vi "top_read_input.vi"(8 "error in (no error)":errorcluster, 10 "Dynamic data":T1, 11 "Input parameters":T2={"Measurement type"=enum."Debug", "Sensor type"=enum."HPK_8in_256", "Identifier"="test.txt", "Open after execution?"=FALSE, "Plot after execution?"=FALSE, "Display channel"=0, "Voltage Delay (s)"=0.5, "Switch Delay (s)"=0.01, "VISA resource name source"="", "VISA resource name DMM"="", "VISA resource name LCR"="", "Compliance  Level (A)"=10.0, "Voltage Limit (V)"=1000.0, "Data storage location"="", "Scan voltages"="", "Use source as DMM?"=FALSE, "LCR signal frequenzy (Hz)"=10.0, "DMM device"=enum."Keithley2001", "Sampling number"=1, "Use env. sensors on"=enum."Sensirion sht1x/7x", "Switchboard Handle"=0, "Use Switchboard"=FALSE, "LCR signal voltage (V)"=10000.0, "Repeat"=1, "Scan voltages IV"="", "Scan voltages CV"="", "Hex pad numbers?"=FALSE, "Set measurement type"=enum."Debug", "Custom pad scan"="", "IV voltage Delay (s)"=0.5, "CV voltage Delay (s)"=0.5, "Needle measurement?"=FALSE, "Comments"="test.txt", "LCR signal frequenzy (kHz)"=10.0, "Compliance  Level (uA)"=10.0, "Open Correction Array"=array2304x3[6912 elements], "Current set voltage"=0.0, "Last set voltage"=0.0, "Current channel"=0, "Last OpenCorrection index"=-1, "Total curr/vltg every x steps"=10, "Current channel iteration"=0, "No CV corrections"=FALSE, "Mapfile"="", "Corrfile"="", "IV voltage file"=path "", "CV voltage file"=path "", "IV Switch Delay (s)"=0.01, "CV Switch Delay (s)"=0.01, "Invert polarity"=FALSE, "Set debug dirs"=FALSE, "Is n on p"=FALSE} {"CV Switch Delay (s)" format="%#_13g"; "IV Switch Delay (s)" format="%#_13g"; "Last set voltage" format="%#_13g"; "Current set voltage" format="%#_13g"; "CV voltage Delay (s)" format="%#_13g"; "IV voltage Delay (s)" format="%#_13g"; "Voltage Limit (V)" format="%#_13g"; "Voltage Delay (s)" format="%#_13g"; "Switch Delay (s)" format="%#_13g"}) -> (0 "error out":errorcluster, 2 "Dynamic data":T1, 3 "Input parameters":T2={"Measurement type"=enum."Debug", "Sensor type"=enum."HPK_8in_256", "Identifier"="test.txt", "Open after execution?"=FALSE, "Plot after execution?"=FALSE, "Display channel"=0, "Voltage Delay (s)"=0.5, "Switch Delay (s)"=0.01, "VISA resource name source"="", "VISA resource name DMM"="", "VISA resource name LCR"="", "Compliance  Level (A)"=10.0, "Voltage Limit (V)"=1000.0, "Data storage location"="", "Scan voltages"="", "Use source as DMM?"=FALSE, "LCR signal frequenzy (Hz)"=10.0, "DMM device"=enum."Keithley2001", "Sampling number"=1, "Use env. sensors on"=enum."Sensirion sht1x/7x", "Switchboard Handle"=0, "Use Switchboard"=FALSE, "LCR signal voltage (V)"=10000.0, "Repeat"=1, "Scan voltages IV"="", "Scan voltages CV"="", "Hex pad numbers?"=FALSE, "Set measurement type"=enum."Debug", "Custom pad scan"="", "IV voltage Delay (s)"=0.5, "CV voltage Delay (s)"=0.5, "Needle measurement?"=FALSE, "Comments"="test.txt", "LCR signal frequenzy (kHz)"=10.0, "Compliance  Level (uA)"=10.0, "Open Correction Array"=array2304x3[6912 elements], "Current set voltage"=0.0, "Last set voltage"=0.0, "Current channel"=0, "Last OpenCorrection index"=-1, "Total curr/vltg every x steps"=10, "Current channel iteration"=0, "No CV corrections"=FALSE, "Mapfile"="", "Corrfile"="", "IV voltage file"=path "", "CV voltage file"=path "", "IV Switch Delay (s)"=0.01, "CV Switch Delay (s)"=0.01, "Invert polarity"=FALSE, "Set debug dirs"=FALSE, "Is n on p"=FALSE} {"CV Switch Delay (s)" format="%#_13g"; "IV Switch Delay (s)" format="%#_13g"; "Last set voltage" format="%#_13g"; "Current set voltage" format="%#_13g"; "CV voltage Delay (s)" format="%#_13g"; "IV voltage Delay (s)" format="%#_13g"; "Voltage Limit (V)" format="%#_13g"; "Voltage Delay (s)" format="%#_13g"; "Switch Delay (s)" format="%#_13g"})   [LabVIEW 2016]
doc: "Processes the user input to generate names and constants to be used during program execution."
uses:
  input_params.ctl
  data_dynamic.ctl
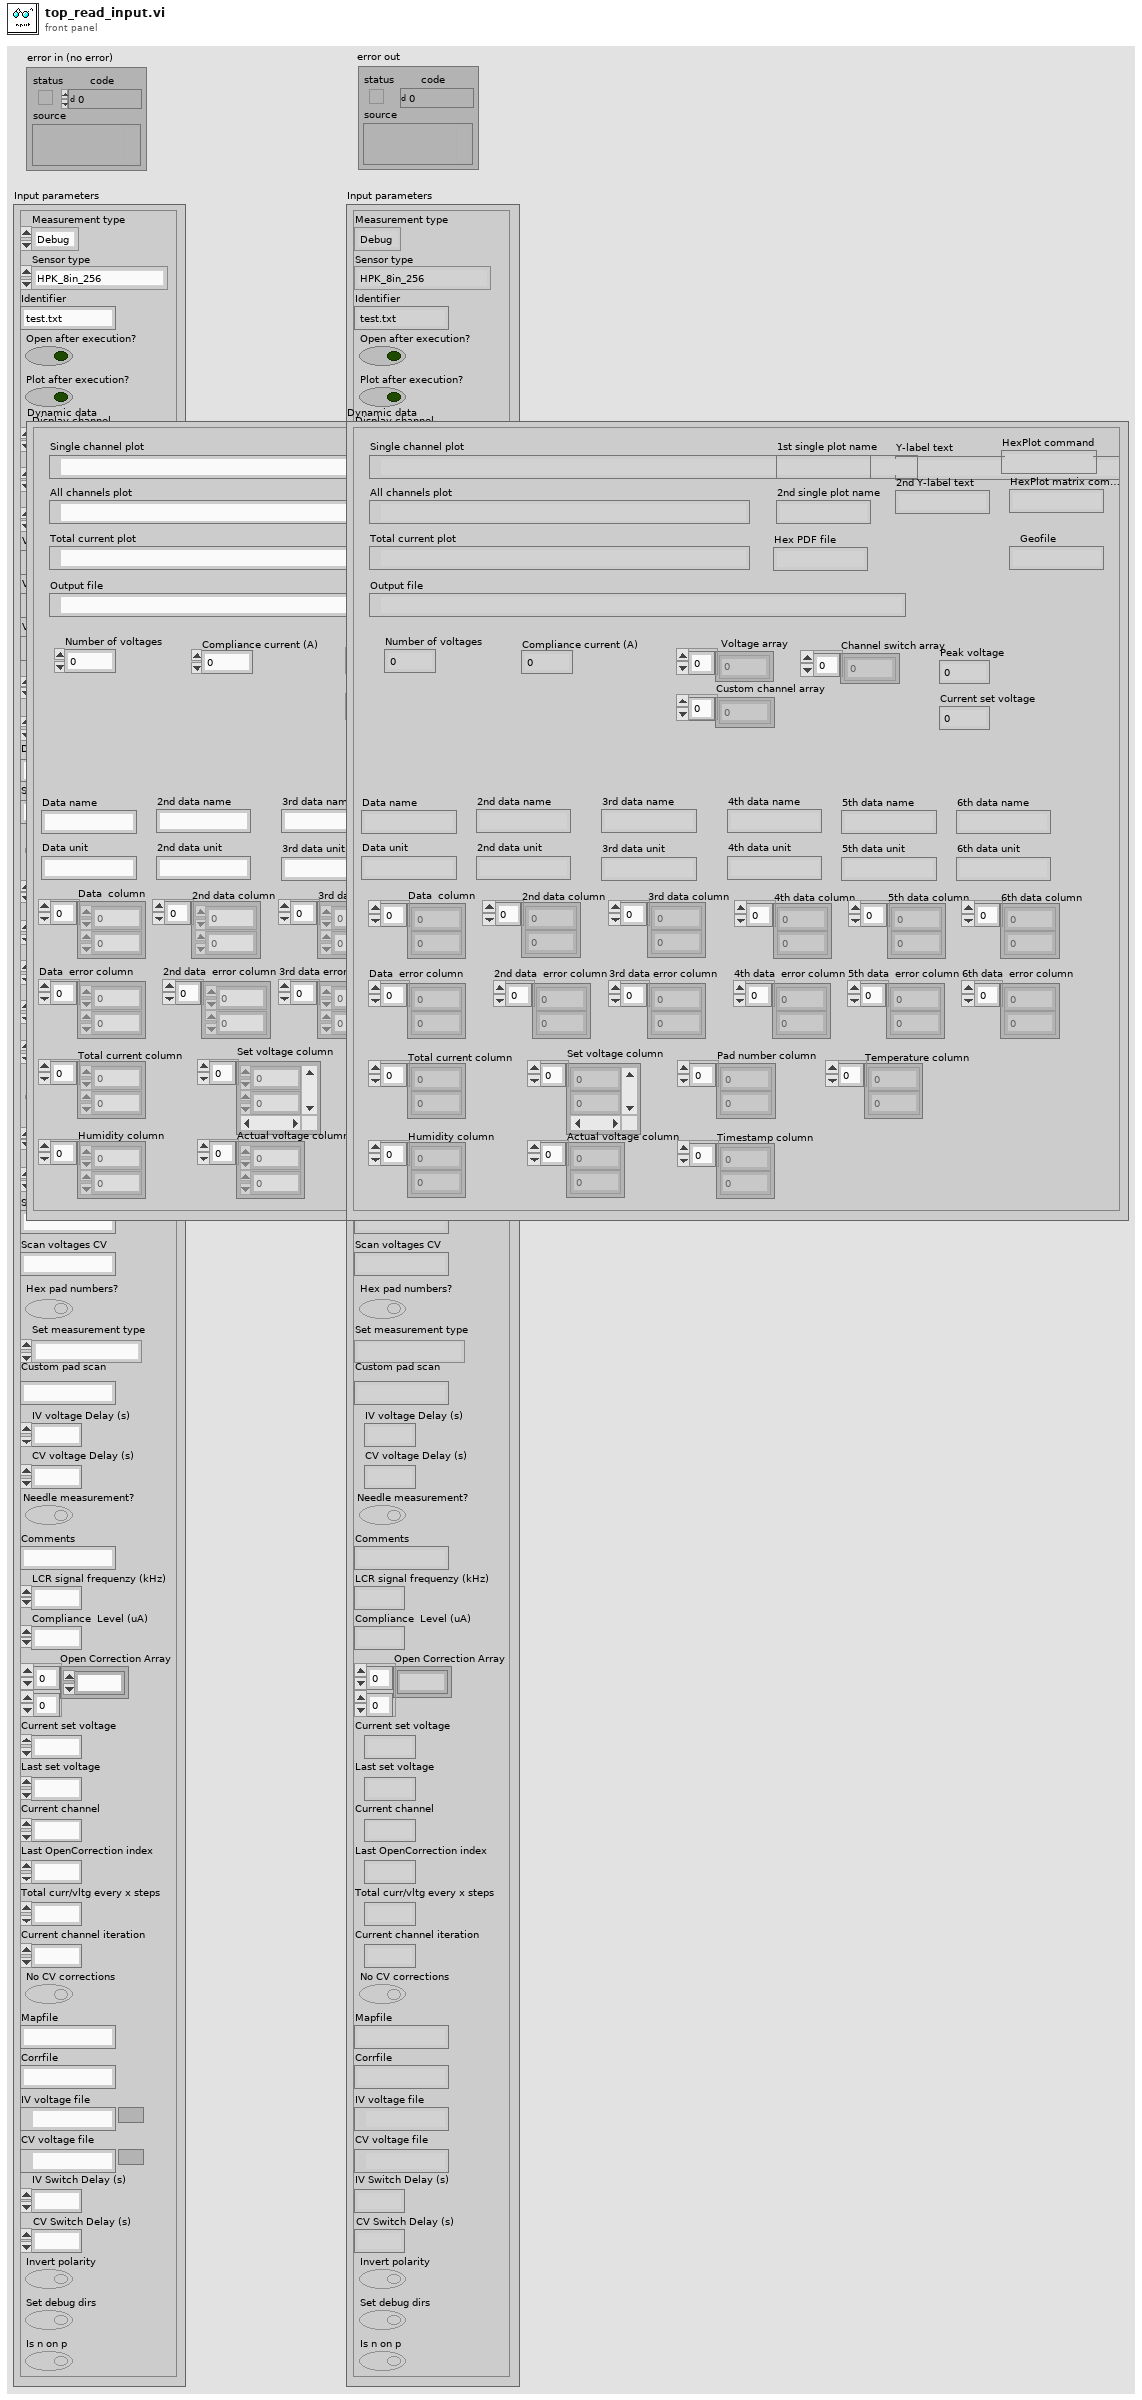
[diagram p1: front panel]
types:
  T1 = typedef "data_dynamic.ctl" = cluster{"Output file":path, "Y-label text":string, "Current set voltage":dbl, "Set voltage column":dbl[], "Pad number column":dbl[], "Data  column":dbl[], "Number of voltages":i32, "Compliance current (A)":dbl, "Geofile":string, "Peak voltage":dbl, "Hex PDF file":string, "Voltage array":dbl[], "Total current column":dbl[], "Timestamp column":dbl[], "Data name":string, "Data unit":string, "2nd data column":dbl[], "2nd data name":string, "2nd data unit":string, "3rd data column":dbl[], "4th data column":dbl[], "3rd data name":string, "3rd data unit":string, "4th data name":string, "4th data unit":string, "Actual voltage column":dbl[], "2nd Y-label text":string, "Single channel plot":path, "Temperature column":dbl[], "Humidity column":dbl[], "Channel switch array":i32[], "1st single plot name":string, "2nd single plot name":string, "All channels plot":path, "HexPlot command":string, "Custom channel array":i32[], "Data  error column":dbl[], "2nd data  error column":dbl[], "3rd data error column":dbl[], "4th data  error column":dbl[], "Total current plot":path, "5th data column":dbl[], "5th data  error column":dbl[], "6th data column":dbl[], "6th data  error column":dbl[], "5th data name":string, "5th data unit":string, "6th data name":string, "6th data unit":string, "HexPlot matrix command":string}
  T2 = typedef "input_params.ctl" = cluster{"Measurement type":enum16{"IV", "CV", "Debug", "Test_contact"}, "Sensor type":enum16{"HPK_6in_135", "HPK_8in_256", "IFX_8in_256", "Diode", "HPK_6in_256", "Full matrix"}, "Identifier":string, "Open after execution?":bool, "Plot after execution?":bool, "Display channel":i32, "Voltage Delay (s)":dbl, "Switch Delay (s)":dbl, "VISA resource name source":refnum<visa-resource-name>, "VISA resource name DMM":refnum<visa-resource-name>, "VISA resource name LCR":refnum<visa-resource-name>, "Compliance  Level (A)":dbl, "Voltage Limit (V)":dbl, "Data storage location":string, "Scan voltages":string, "Use source as DMM?":bool, "LCR signal frequenzy (Hz)":dbl, "DMM device":enum16{"Keithley2001", "Keithley2450", "Keithley2410", "Keithley6487"}, "Sampling number":i32, "Use env. sensors on":enum16{"Sensirion sht1x/7x", "Switch Matrix", "Probecard"}, "Switchboard Handle":u32, "Use Switchboard":bool, "LCR signal voltage (V)":dbl, "Repeat":i32, "Scan voltages IV":string, "Scan voltages CV":string, "Hex pad numbers?":bool, "Set measurement type":enum16{"IV", "CV", "Debug", "Test_contact", "IV+CV"}, "Custom pad scan":string, "IV voltage Delay (s)":dbl, "CV voltage Delay (s)":dbl, "Needle measurement?":bool, "Comments":string, "LCR signal frequenzy (kHz)":dbl, "Compliance  Level (uA)":dbl, "Open Correction Array":dbl[][], "Current set voltage":dbl, "Last set voltage":dbl, "Current channel":i32, "Last OpenCorrection index":i32, "Total curr/vltg every x steps":i32, "Current channel iteration":i32, "No CV corrections":bool, "Mapfile":string, "Corrfile":string, "IV voltage file":path, "CV voltage file":path, "IV Switch Delay (s)":dbl, "CV Switch Delay (s)":dbl, "Invert polarity":bool, "Set debug dirs":bool, "Is n on p":bool}
  T3 = enum16{"HPK_6in_135", "HPK_8in_256", "IFX_8in_256", "Diode", "HPK_6in_256", "Full matrix"}
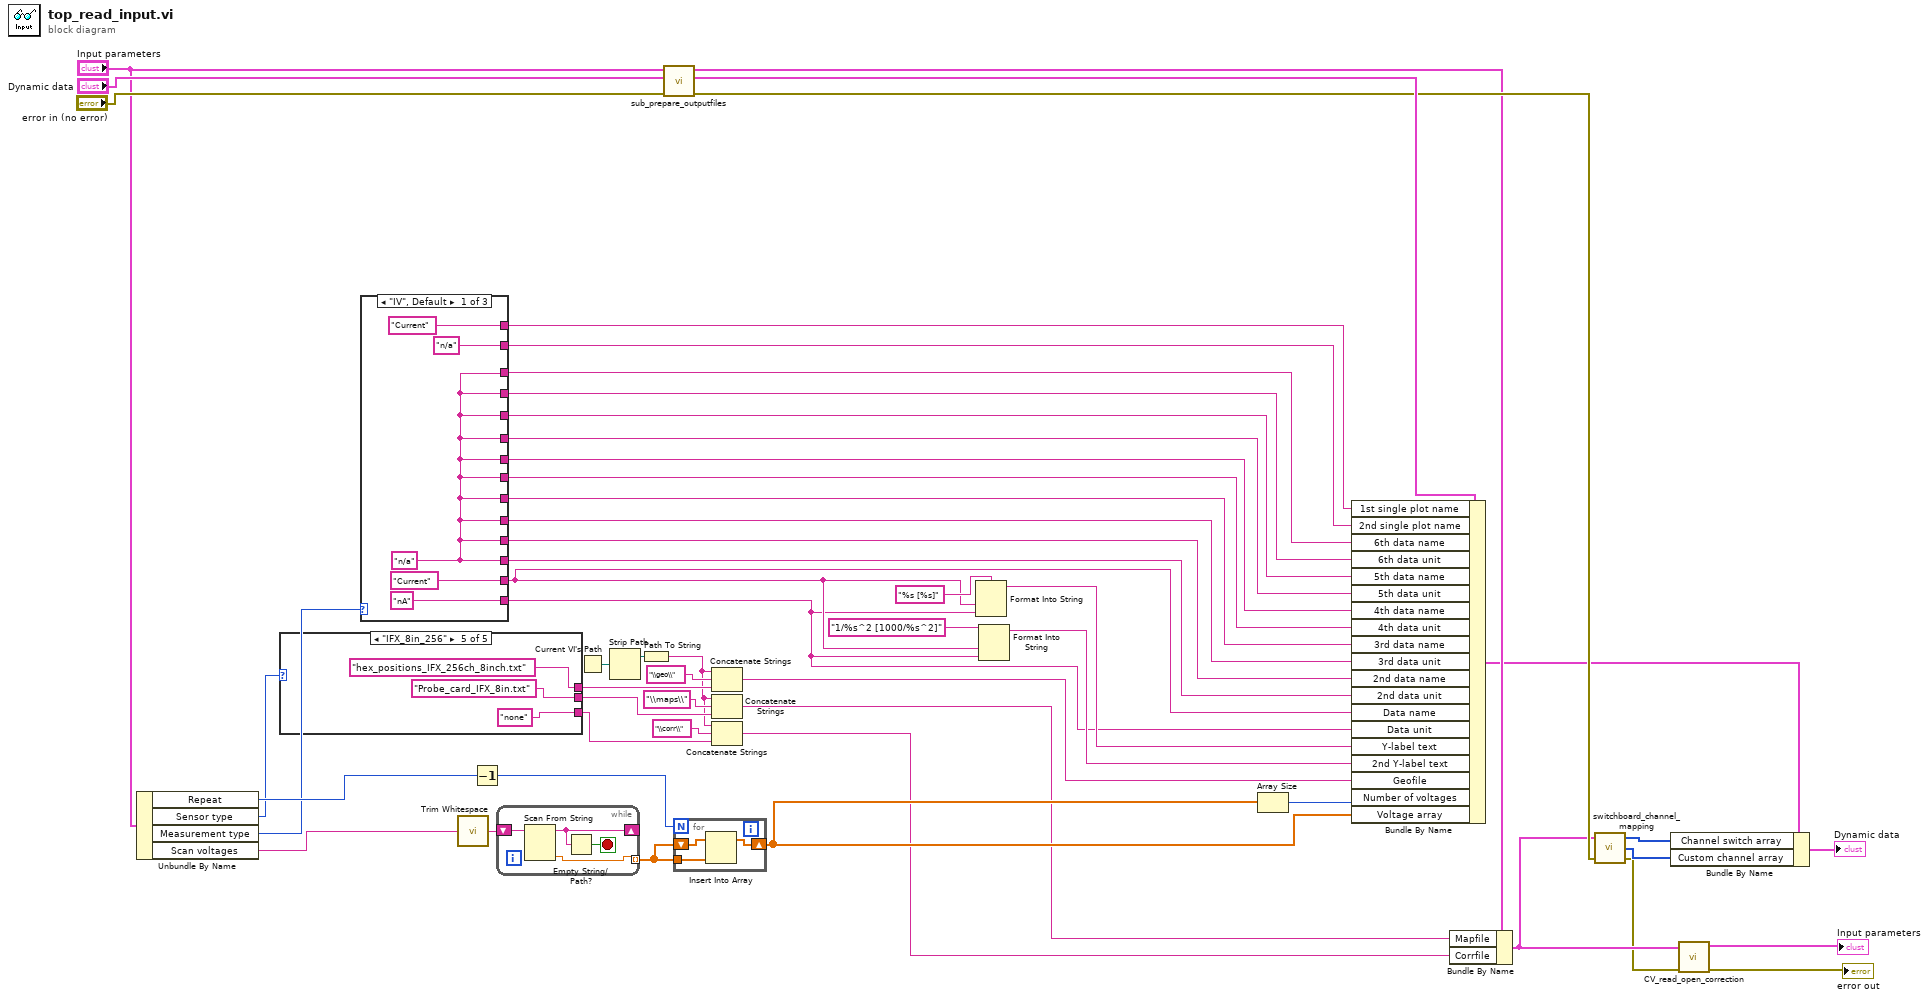
[diagram p0: block diagram]
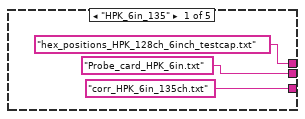
[diagram p2: hidden frame]
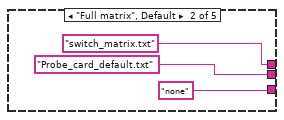
[diagram p3: hidden frame]
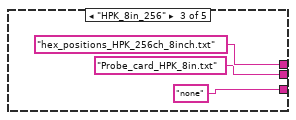
[diagram p4: hidden frame]
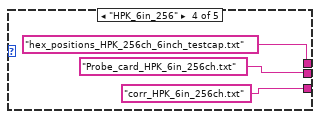
[diagram p5: hidden frame]
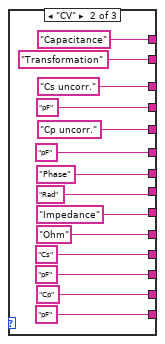
[diagram p6: hidden frame]
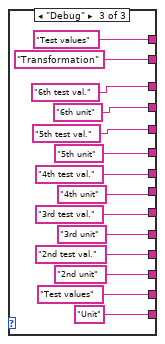
[diagram p7: hidden frame]
diagram:
  n1 = Unbundle By Name("Input parameters") -> ("Repeat"=w38:i32, "Sensor type"=w18:T3, "Measurement type"=w29:enum16{"IV", "CV", "Debug", "Test_contact"}, "Scan voltages"=w33:string)
  n2 = case shown="\"IFX_8in_256\"" w18 {
    tunnel: ["hex_positions_HPK_128ch_6inch_testcap.txt" "switch_matrix.txt" ("name or relative path") "hex_positions_HPK_256ch_8inch.txt" ("name or relative path") "hex_positions_HPK_256ch_6inch_testcap.txt" ("name or relative path") "hex_positions_IFX_256ch_8inch.txt" ("name or relative path")] -> w53
    tunnel: ["Probe_card_HPK_6in.txt" "Probe_card_default.txt" ("name or relative path") "Probe_card_HPK_8in.txt" ("name or relative path") "Probe_card_HPK_6in_256ch.txt" ("name or relative path") "Probe_card_IFX_8in.txt" ("name or relative path")] -> w16
    tunnel: ["corr_HPK_6in_135ch.txt" ("name or relative path") "none" ("name or relative path") "none" ("name or relative path") "corr_HPK_6in_256ch.txt" ("name or relative path") "none" ("name or relative path")] -> w7
    frame "HPK_6in_135" {
    }
    frame "Full matrix", Default {
    }
    frame "HPK_8in_256" {
    }
    frame "HPK_6in_256" {
    }
    frame "IFX_8in_256" {
    }
  }
  n3 = case shown="\"IV\", Default" w29 {
    tunnel: ["Current" "Cp" "Test values"] -> w41
    tunnel: ["nA" "pF" "Unit"] -> w28
    tunnel: [w69 "Cs" "2nd test val."] -> w24
    tunnel: [w69 "pF" "2nd unit"] -> w47
    tunnel: [w69 "Ohm" "3rd unit"] -> w46
    tunnel: [w69 "Impedance" "3rd test val."] -> w45
    tunnel: [w69 "Rad" "4th unit"] -> w44
    tunnel: [w69 "Phase" "4th test val."] -> w43
    tunnel: ["Current" "Capacitance" "Test values"] -> w34
    tunnel: ["n/a" "Transformation" "Transformation"] -> w35
    tunnel: [w69 "pF" "5th unit"] -> w22
    tunnel: [w69 "Cp uncorr." "5th test val."] -> w21
    tunnel: [w69 "pF" "6th unit"] -> w20
    tunnel: [w69 "Cs uncorr." "6th test val."] -> w19
    frame "IV", Default {
      w69 = "n/a"
    }
    frame "CV" {
    }
    frame "Debug" {
    }
  }
  n4 = call <vilib>:"Trim Whitespace.vi"("string"=w33) -> ("trimmed string"=w51:string)  [unwired: 1 in]
  n5 = Decrement(x=w38) -> (x-1=w36:i32)
  n6 = while {
    shift-right: [w104] -> _
    shift-left: w51 -> [w105]
    tunnel: [w102] -> w37 mode=indexing
    stop <- w103 stop-if-true
    n7 = Scan From String(input string=w105) -> (remaining string=w104:string, output 1=w102:dbl)  [unwired: 4 in, 2 out]
    n8 = Empty String/Path?(string/path=w104) -> (empty?=w103:bool)
  }
  n9 = Current VI's Path() -> (path=w50:path)
  n10 = Strip Path(path=w50) -> (stripped path=w49:path)  [unwired: 1 out]
  n11 = Path To String(path=w49) -> (string=w9:string)
  n12 = call "sub_prepare_outputfiles.vi"("error in"="error in (no error)", "Dynamic data in"="Dynamic data", "Input parameters"="Input parameters") -> ("error out"=w26:errorcluster, "Dynamic data out"=w30:T1, "Input parameters out"=w25:T2)  [unwired: 6 in]
  n13 = for {
    N: w36 -> [_]
    tunnel: w37 -> [w107]
    shift-right: [w106] -> w23
    shift-left: w37 -> [w108]
    n14 = Insert Into Array(array=w108, new element=w107) -> (w106:dbl[])  [unwired: 1 in]
  }
  n15 = Concatenate Strings(w9, "\\geo\\" ("string"), w53) -> (w27:string)
  n16 = Concatenate Strings(w9, "\\maps\\" ("string"), w16) -> (w14:string)
  n17 = Concatenate Strings(w9, "\\corr\\" ("string"), w7) -> (w6:string)
  n18 = Format Into String(format string="%s [%s]", w41, w28) -> (resulting string=w39:string)  [unwired: 2 in, 1 out]
  n19 = Format Into String(format string="1/%s^2 [1000/%s^2]", w41, w28) -> (resulting string=w40:string)  [unwired: 2 in, 1 out]
  n20 = Array Size(array=w23) -> (size(s)=w52:i32)
  n21 = Bundle By Name(cluster=w30, "1st single plot name"=w34, "2nd single plot name"=w35, "6th data name"=w19, "6th data unit"=w20, "5th data name"=w21, "5th data unit"=w22, "4th data name"=w43, "4th data unit"=w44, "3rd data name"=w45, "3rd data unit"=w46, "2nd data name"=w24, "2nd data unit"=w47, "Data name"=w41, "Data unit"=w28, "Y-label text"=w39, "2nd Y-label text"=w40, "Geofile"=w27, "Number of voltages"=w52, "Voltage array"=w23) -> (w12:T1)
  n22 = Bundle By Name(cluster=w25, "Mapfile"=w14, "Corrfile"=w6) -> (w5:T2)
  n23 = call "switchboard_channel_mapping.vi"("error in"=w26, "Input parameters"=w5) -> ("error out"=w3:errorcluster, "Custom pad array"=w10:i32[], "Channel array"=w13:i32[])  [unwired: 1 in]
  n24 = Bundle By Name(cluster=w12, "Channel switch array"=w13, "Custom channel array"=w10) -> (→"Dynamic data":T1)
  n25 = call "CV_read_open_correction.vi"("error in"=w3, "Input parameters in"=w5) -> ("error out"=→"error out":errorcluster, "Input parameters out"=→"Input parameters":T2)  [unwired: 8 in]
